vi "GEOM_SortAmplifiers.vi"(10 "amplifiers":T1[](array[typedef]) {"fliped" items=["none", "horizontal", "vertical"]; "type" items=["LL", "LR", "UL", "UR"]}) -> (2 "sorted amplifiers":T1[](array[typedef]) {"fliped" items=["none", "horizontal", "vertical"]; "type" items=["LL", "LR", "UL", "UR"]})   [LabVIEW 2016]
uses:
  GEOM_Amplifier.ctl
  GEOM_AmpType.ctl
  GEOM_ROI.ctl
  GEOM_Coords.ctl
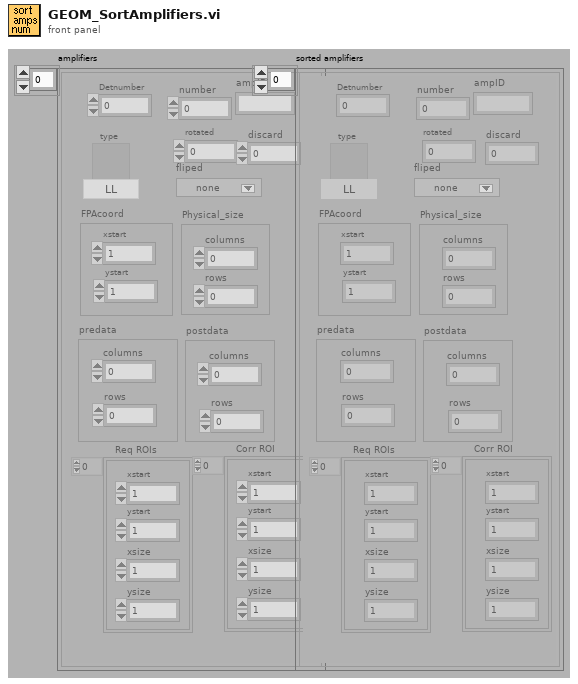
[diagram p1: front panel]
types:
  T1 = typedef "GEOM_Amplifier.ctl" = cluster{"number":i32, "type":T2, "rotated":i16, "fliped":u16, "FPAcoord":cluster{"xstart":i32, "ystart":i32}, "Physical_size":cluster{"columns":i32, "rows":i32}, "predata":cluster{"columns":i32, "rows":i32}, "postdata":cluster{"columns":i32, "rows":i32}, "Req ROIs":T3, "Corr ROI":T3, "Detnumber":i32, "ampID":string, "discard":i32}
  T2 = typedef "GEOM_AmpType.ctl" = u16
  T3 = typedef "GEOM_ROI.ctl" = T4[]
  T4 = typedef "GEOM_Coords.ctl" = cluster{"xstart":u32, "ystart":u32, "xsize":u32, "ysize":u32}
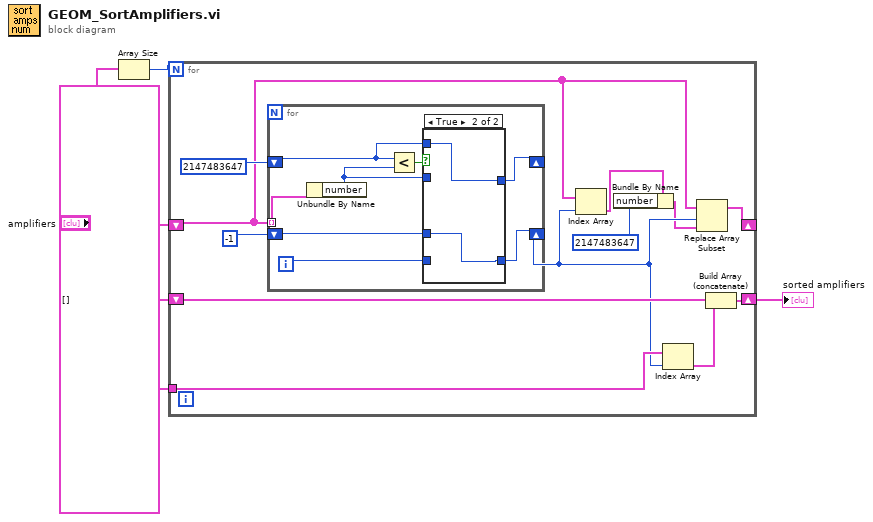
[diagram p0: block diagram]
diagram:
  n1 = Array Size(array="amplifiers") -> (size(s)=w3:i32)
  n2 = for {
    N: w3 -> [_]
    shift-right: [w10] -> _
    shift-left: "amplifiers" -> [w8]
    shift-right: [w12] -> w2
    shift-left: T1[] [] -> [w11]
    tunnel: "amplifiers" -> [w14]
    n3 = for {
      shift-right: [w20] -> _
      shift-left: 2147483647 -> [w19]
      tunnel: w8 -> [w24] mode=indexing
      shift-right: [w18] -> w9
      shift-left: -1 -> [w17]
      i -> [w22]
      n4 = Unbundle By Name(w24) -> ("number"=w21:i32)
      n5 = Less?(x=w19, y=w21) -> (x < y?=w23:bool)
      n6 = case shown="True" w23 {
        tunnel: w22 -> [w25 _]
        tunnel: w21 -> [w26 _]
        tunnel: [w26 w28] -> w20
        tunnel: w19 -> [_ w28]
        tunnel: [w25 w27] -> w18
        tunnel: w17 -> [_ w27]
        frame False {
        }
        frame True {
        }
      }
    }
    n7 = Index Array(array=w8, index=w9) -> (element=w7:T1)
    n8 = Bundle By Name(cluster=w7, "number"=2147483647) -> (w6:T1)
    n9 = Index Array(array=w14, index=w9) -> (element=w13:T1)
    n10 = Replace Array Subset(array=w8, new element=w6, index=w9) -> (w10:T1[])
    n11 = Build Array (concatenate)(w11, w13) -> (w12:T1[])
  }
  "sorted amplifiers" <- w2
